vi "Get Extended Selection.vi"(8 "error in (no error)":errorcluster, 10 "Selected":i16[](array[numeric]), 11 "Shapes":refnum<data-value>[](array[refnum])) -> (0 "error out":errorcluster, 2 "Ext. Selection":i32[](array[numeric]), 3 "Shapes out":refnum<data-value>[](array[refnum]))   [LabVIEW 2015, in "LV Image Editor Framework.lvlib" / "Image Editor Handler.lvclass"]
uses:
  Image Editor Handler.lvclass
  Forms/Shape/Shape.lvclass
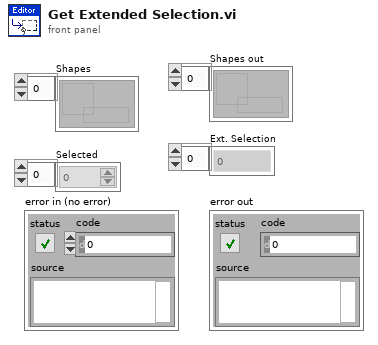
[diagram p1: front panel]
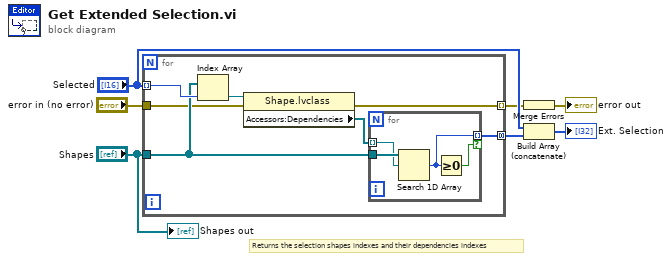
[diagram p0: block diagram]
diagram:
  # "Returns the selection shapes indexes and their dependencies indexes"
  n1 = for {
    tunnel: "Selected" -> [w14] mode=indexing
    tunnel: "Shapes" -> [w12]
    tunnel: [w10] -> w5 mode=concatenating
    tunnel: "error in (no error)" -> [w9]
    tunnel: [w8] -> w3 mode=indexing
    n2 = Index Array(array=w12, index=w14) -> (element=w13:refnum<data-value>)
    n3 = property class="Shape.lvclass"(reference=w13, error in=w9) -> (error out=w8:errorcluster, "Accessors:Dependencies"=w11:refnum<data-value>[])  [unwired: 1 out]
    n4 = for {
      tunnel: w12 -> [w18]
      tunnel: w11 -> [w17] mode=indexing
      tunnel: [w16] -> w10 mode=indexing if=w15
      n5 = Search 1D Array(1D array=w18, element=w17) -> (index of element=w16:i32)  [unwired: 1 in]
      n6 = Greater Or Equal To 0?(x=w16) -> (x >= 0?=w15:bool)
    }
  }
  n7 = Merge Errors(w3) -> (→"error out":errorcluster)
  n8 = Build Array (concatenate)("Selected", w5) -> (→"Ext. Selection":i32[])
  "Shapes out" <- "Shapes"
